vi "Read Measurement Edge.vi"(8 "error in":errorcluster, 11 "period measurement channel in":refnum<class "Period Measurement Channel.lvclass">) -> (0 "error out":errorcluster, 2 "measurement edge":T1, 3 "period measurement channel out":refnum<class "Period Measurement Channel.lvclass">)   [LabVIEW 2017, in "Period Measurement Channel.lvclass"]
uses:
  Period Measurement Channel.lvclass
  Measurement Edge.ctl
  Period Measurement Channel.lvclass/Period Measurement Channel.ctl
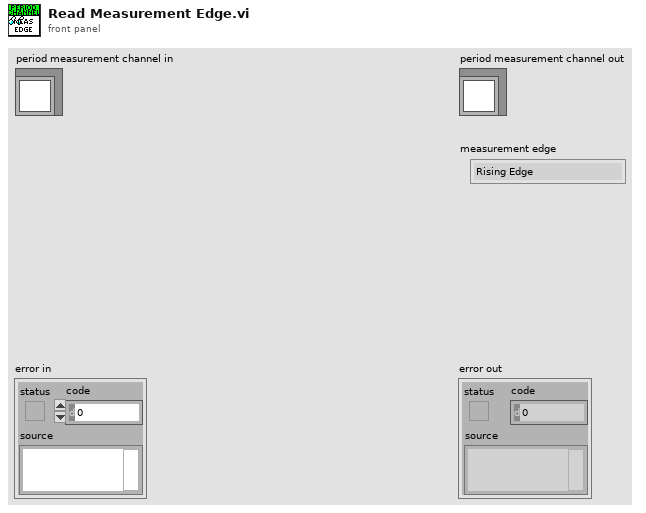
[diagram p1: front panel]
types:
  T1 = typedef "Period Measurement Channel.lvclass/Measurement Edge.ctl" = enum16{"Rising Edge", "Falling Edge"}
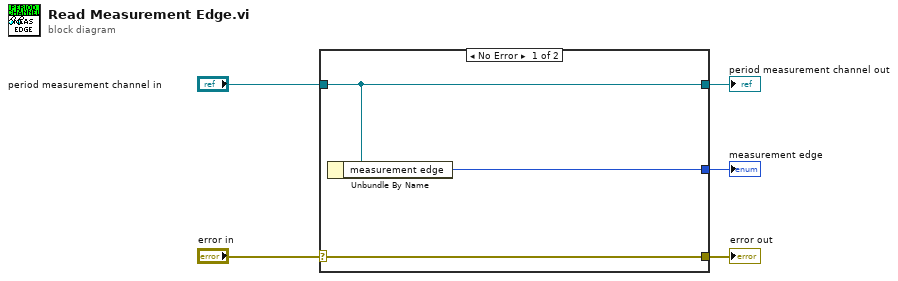
[diagram p0: block diagram]
diagram:
  n1 = case shown="No Error" "error in" {
    selector: "error in" -> [w8 w9]
    tunnel: [w8 w9] -> w4
    tunnel: [w7 w10] -> w2
    tunnel: "period measurement channel in" -> [w7 w10]
    tunnel: [w6 _] -> w1
    frame No Error {
      n2 = Unbundle By Name(w7) -> ("measurement edge"=w6:T1)
    }
    frame Error {
    }
  }
  "error out" <- w4
  "period measurement channel out" <- w2
  "measurement edge" <- w1
